vi "AutoDropStack.vi"() -> (0 "Done?":bool)   [LabVIEW 2014]
uses:
  Robot Global Data.vi
  Elevator/Elevator Command.ctl
  Common Code/Elevator Mode.ctl
  Elevator/Elevator Control Command.ctl
  Common Code/Elevator Idle Mode.ctl
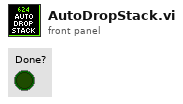
[diagram p1: front panel]
types:
  T1 = typedef "Elevator Command.ctl" = enum16{"Idle", "Load 1", "Load 2", "Load 3", "Drop Stack", "Eject Stack", "Untip Trashcan", "Load Trashcan", "HP Load"}
  T2 = typedef "Elevator Mode.ctl" = enum16{"Manual", "Safe", "Auto"}
  T3 = typedef "Elevator Control Command.ctl" = cluster{"Command":T1, "Manual Motor Out":dbl, "Manual Eject Piston":bool, "Mode":T2, "Override Limits":bool, "Manual Stabilizer":bool, "Manual Finger":bool, "Store Trashcan?":bool, "Hold Low?":bool, "Idle Mode":T4, "HP Load":bool}
  T4 = typedef "Elevator Idle Mode.ctl" = enum16{"Load 1", "Load 2", "Load 3", "Load Can", "Untip Can", "Step Load", "Drop Stack"}
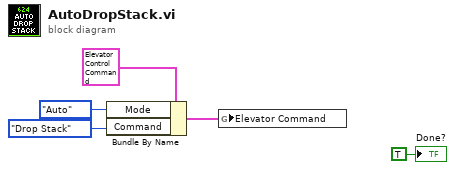
[diagram p0: block diagram]
diagram:
  n1 = Bundle By Name(cluster=T3 {"Command"=enum."Idle", "Manual Motor Out"=0.0, "Manual Eject Piston"=FALSE, "Mode"=enum."Manual", "Override Limits"=FALSE, "Manual Stabilizer"=FALSE, "Manual Finger"=FALSE, "Store Trashcan?"=FALSE, "Hold Low?"=FALSE, "Idle Mode"=enum."Load 1", "HP Load"=FALSE} ("Elevator Command"), "Mode"=Elevator_Mode."Auto", "Command"=Elevator_Command."Drop Stack") -> (w2:T3)
  n2 = global write "Robot Global Data.vi" "Elevator Command"(w2) -> ()
  "Done?" <- TRUE ("Done?")
